vi "Cmd Set Parameter Properties (C).vi"(4 "error in (no error)":errorcluster, 5 "parameter properties":T1, 6 "parameter index":variant, 7 "command reference":T4) -> (0 "error out":errorcluster, 3 "command reference out":T4)   [LabVIEW 2012, in "NI_Database_API_64.lvlib"]
doc: "Sets properties on the object as determined by the inputs. Wire data to the reference and properties inputs to determine the polymorphic instance to use or manually select the instance."
uses:
  NI_Database_API_64.lvlib
  Cmd ObjectReference.ctl
  Cmd Parameter Properties.ctl
  Auxilliary.llb/DB Tools DataTypes.ctl
  Auxilliary.llb/DB Tools Parameter Dir.ctl
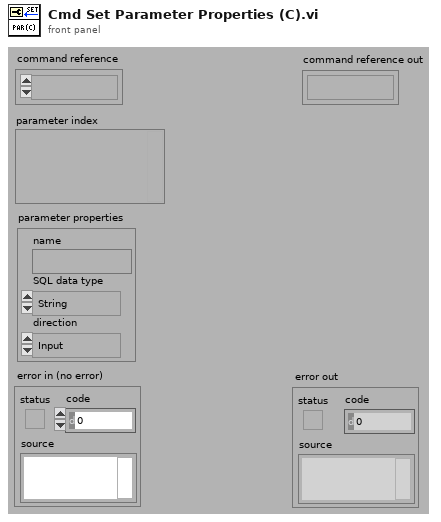
[diagram p1: front panel]
types:
  T1 = typedef "NI_Database_API_64.lvlib/Cmd Parameter Properties.ctl" = cluster{"name":string, "SQL data type":T2, "direction":T3}
  T2 = typedef "NI_Database_API_64.lvlib/DB Tools DataTypes.ctl" = enum16{"String", "Long (I32)", "Single (SGL)", "Double (DBL)", "Date/Time", "Binary"}
  T3 = typedef "NI_Database_API_64.lvlib/DB Tools Parameter Dir.ctl" = enum32{"Input", "Output", "Input/Output", "Return Value"}
  T4 = typedef "NI_Database_API_64.lvlib/Cmd ObjectReference.ctl" = refnum<k1>
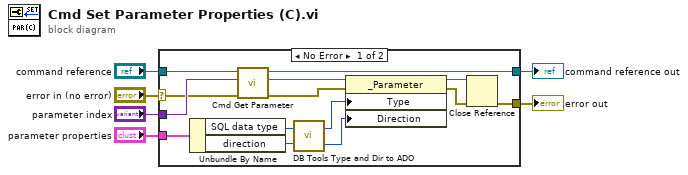
[diagram p0: block diagram]
diagram:
  n1 = case shown="No Error" "error in (no error)" {
    selector: "error in (no error)" -> [w7 w22]
    tunnel: "command reference" -> [w19 w21]
    tunnel: "parameter index" -> [w18 _]
    tunnel: [w17 w21] -> w4
    tunnel: [w14 w22] -> w3
    tunnel: "parameter properties" -> [w13 _]
    frame No Error {
      n2 = Unbundle By Name(w13) -> ("SQL data type"=w12:T2, "direction"=w11:T3)
      n3 = call "Cmd Get Parameter.vi"("error in (no error)"=w7, "parameter index"=w18, "command reference"=w19) -> ("error out"=w15:errorcluster, "ADODB.Parameter"=w16:refnum<k7>, "command reference out"=w17:T4)  [unwired: 2 in]
      n4 = call "DB Tools Type and Dir to ADO.vi"("direction"=w11, "data type"=w12) -> ("ADO direction"=w9:u16, "ADO type"=w10:u16)
      n5 = property class="_Parameter"(reference=w16, error in=w15, "Type"=w10, "Direction"=w9) -> (reference out=w20:refnum<k7>, error out=w8:errorcluster)
      n6 = Close Reference(reference=w20, error in (no error)=w8) -> (error out=w14:errorcluster)
    }
    frame Error {
    }
  }
  "command reference out" <- w4
  "error out" <- w3
